vi "MB_TCP_7051.vi"(5 "Status Reference":T1, 6 "N":i32, 7 "Data Reference":T2, 9 "timeouts":T3={"conn_timeout"=1000, "reconn_timeout"=3000, "N attempt max"=3, "t_reset_TTL"=120000, "write_timeout"=10, "read_timeout"=500, "period"=100} {"t_reset_TTL" min=10 max=240000 step=1; "period" min=10 max=100000 step=1; "read_timeout" min=10 max=60000 step=1; "write_timeout" min=1 max=60000 step=1; "N attempt max" min=1 max=5 step=1; "reconn_timeout" min=10 max=240000 step=1; "conn_timeout" min=10 max=240000}, 10 "write enable":bool=TRUE, 11 "stop":bool) -> (0 "error out":errorcluster, 2 "errors":i32, 3 "Z3":u32)   [LabVIEW 2019, in "MB_TCP1.lvlib"]
uses:
  MB_TCP1.lvlib
  Timer Delay/Timers.lvlib
  NI_modbus_upd/NI_modbus_upd.lvlib
  NI_modbus_upd/MB Modbus Command.ctl
  ICPCON Registers/ICPCON Registers.lvlib
  ICPCON Status/ICPCON Status.lvlib
  Timer Delay/unix time 1ms.vi
  NI_modbus_upd/TCP/TCP.lvclass
  ICPCON Registers/Ctl/ICPCON Data.ctl
  ICPCON Status/Ctl/ICPCON Status.ctl
panel:
  out "stopped":bool
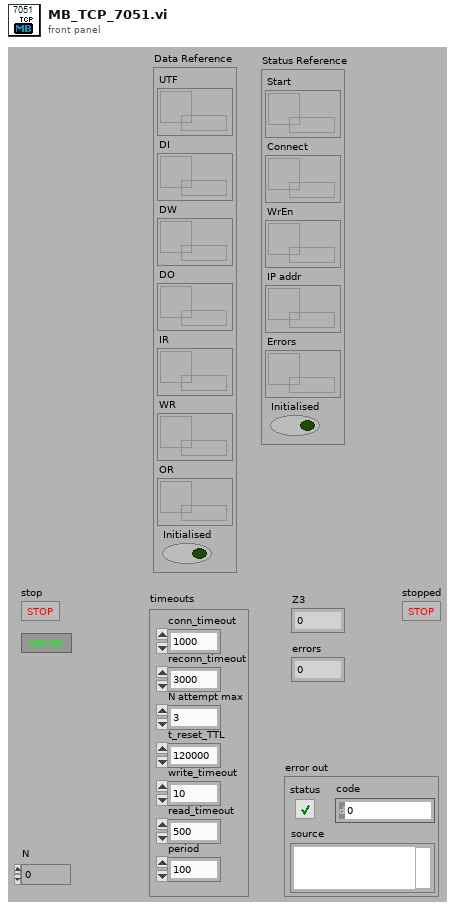
[diagram p1: front panel]
types:
  T1 = typedef "ICPCON Status.lvlib/ICPCON Status.ctl" = cluster{"Start":refnum<data-value>, "Connect":refnum<data-value>, "WrEn":refnum<data-value>, "IP addr":refnum<data-value>, "Errors":refnum<data-value>, "Initialised":bool}
  T2 = typedef "ICPCON Registers.lvlib/ICPCON Data.ctl" = cluster{"UTF":refnum<data-value>, "DI":refnum<data-value>, "DW":refnum<data-value>, "DO":refnum<data-value>, "IR":refnum<data-value>, "WR":refnum<data-value>, "OR":refnum<data-value>, "Initialised":bool}
  T3 = cluster{"conn_timeout":i32, "reconn_timeout":i32, "N attempt max":i32, "t_reset_TTL":i32, "write_timeout":i32, "read_timeout":i32, "period":i32}
  T4 = typedef "NI_modbus_upd.lvlib/MB Modbus Command.ctl" = cluster{"Function Code":u8, "Starting Address":u16, "Quantity":u16, "Data":u16[], "Discrete":bool[]}
  T5 = cluster{"Transaction ID":u16, "Protocol ID":u16, "Length":u16, "Unit ID":u8}
  T6 = cluster{"Remote IP Address":string, "Remote Port":u16}
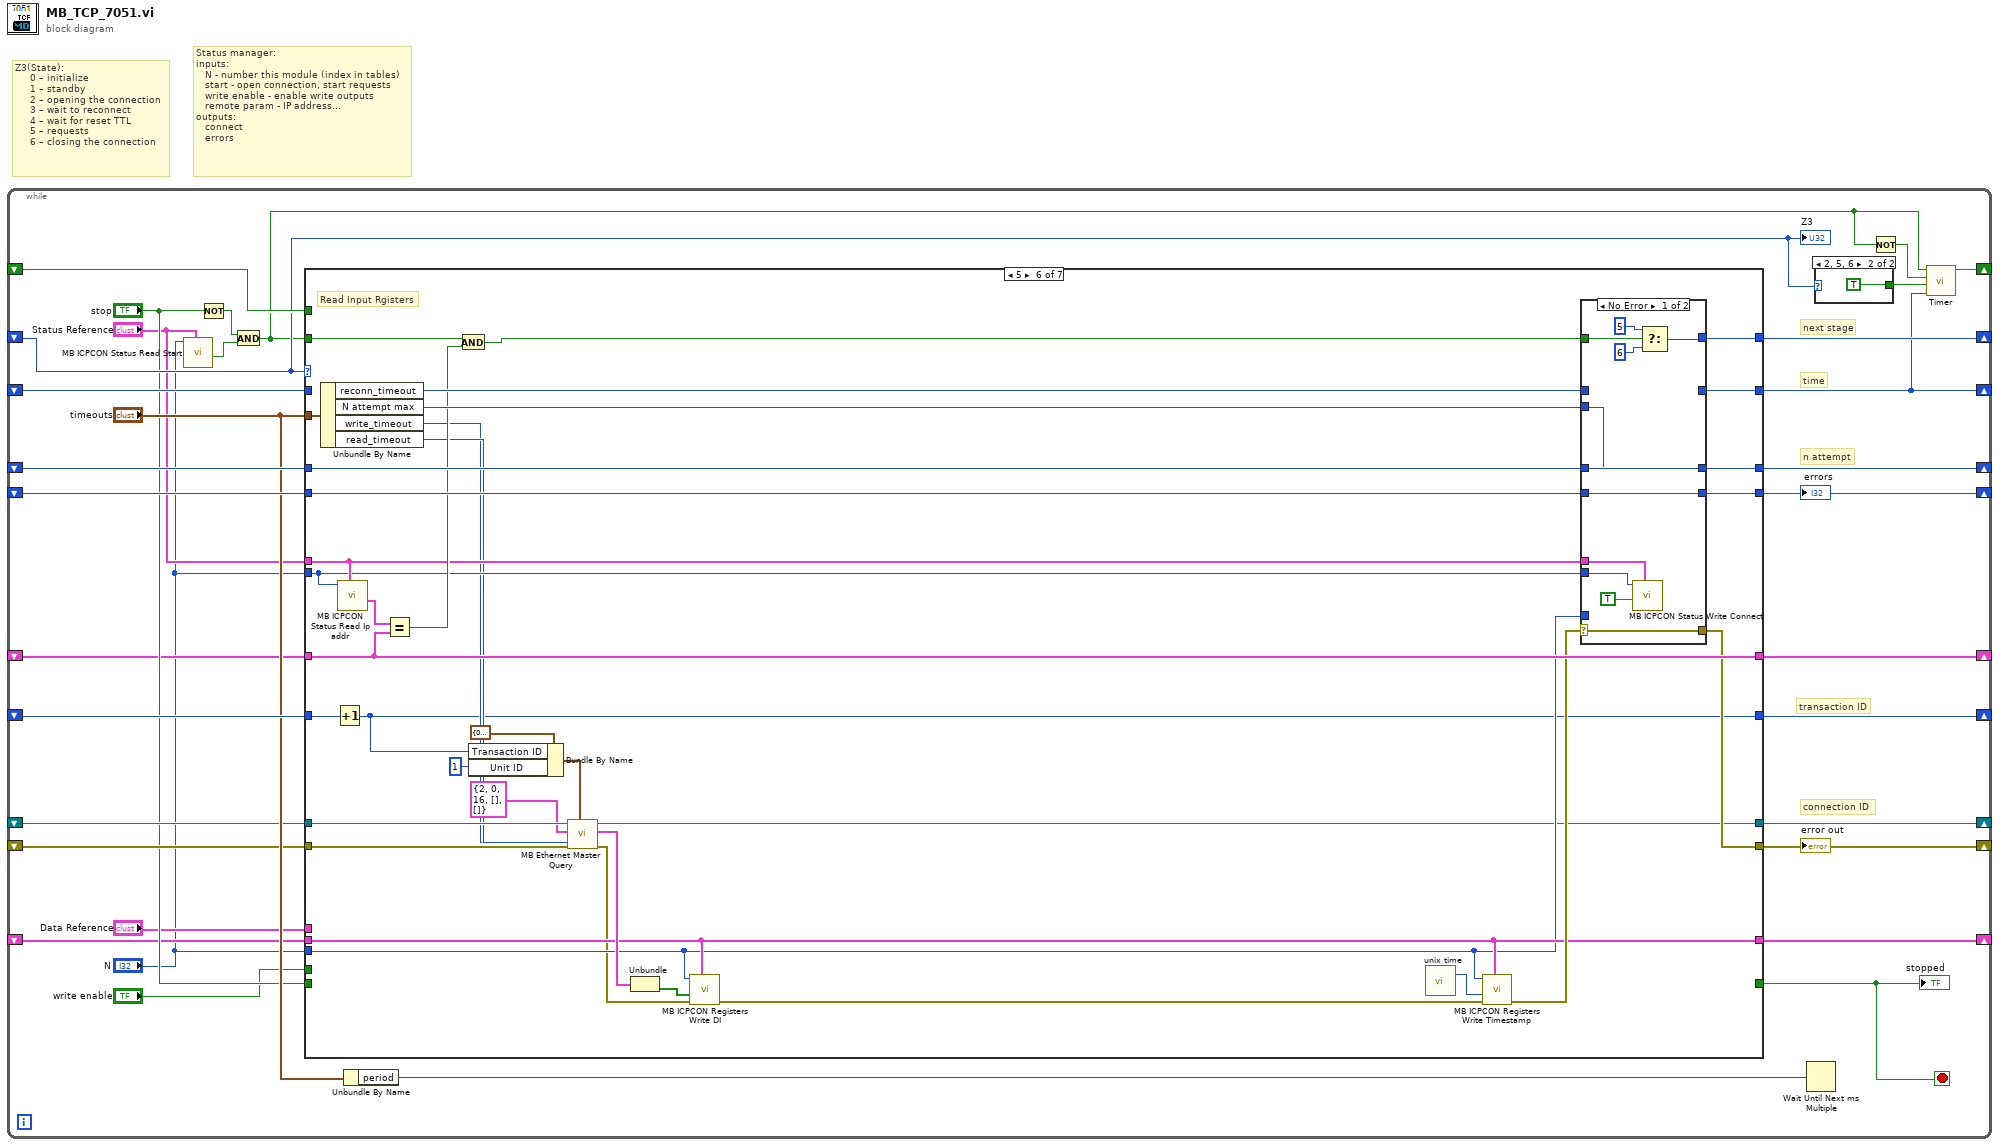
[diagram p0: block diagram]
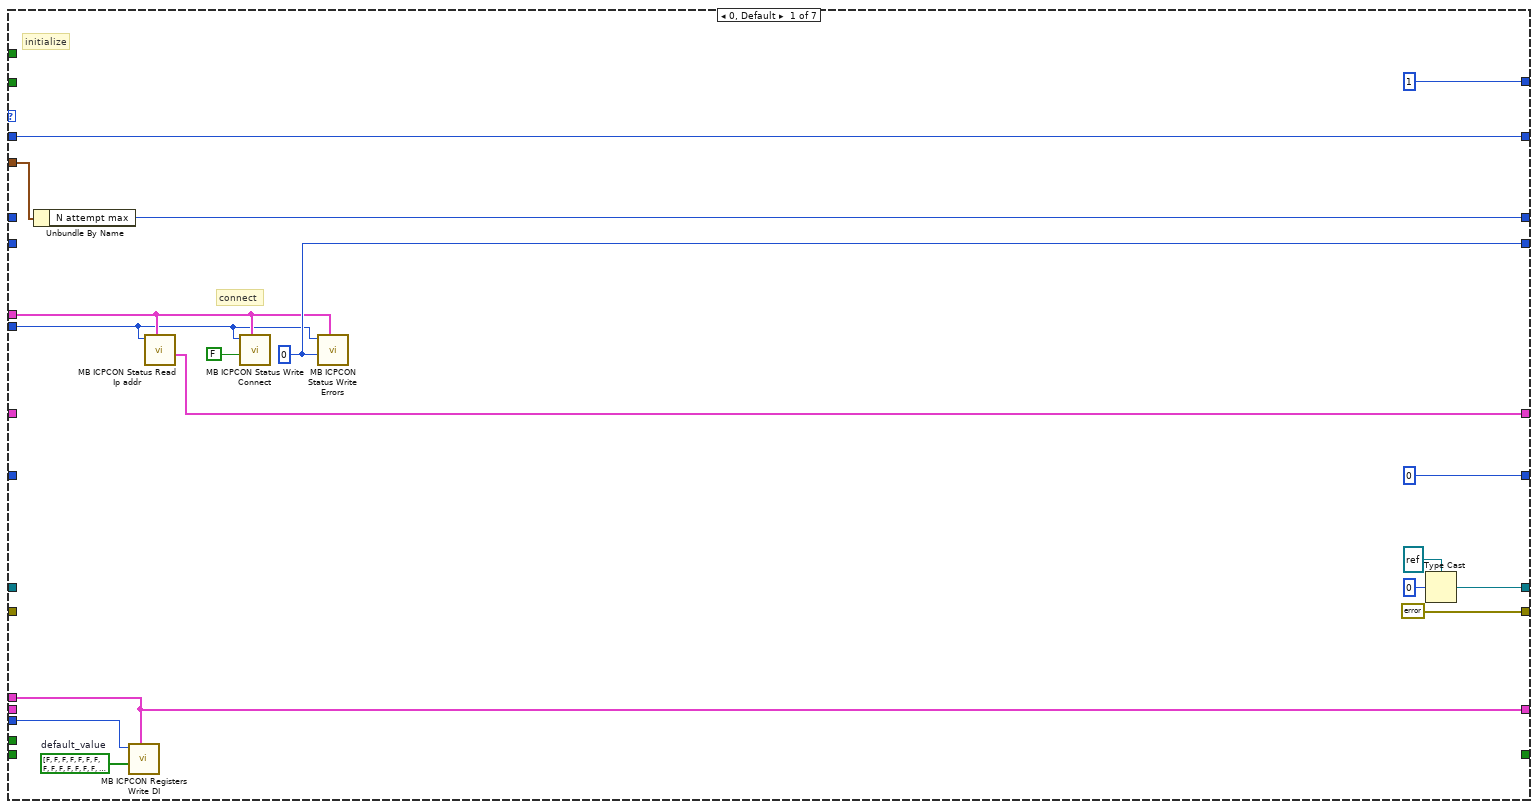
[diagram p2: hidden frame]
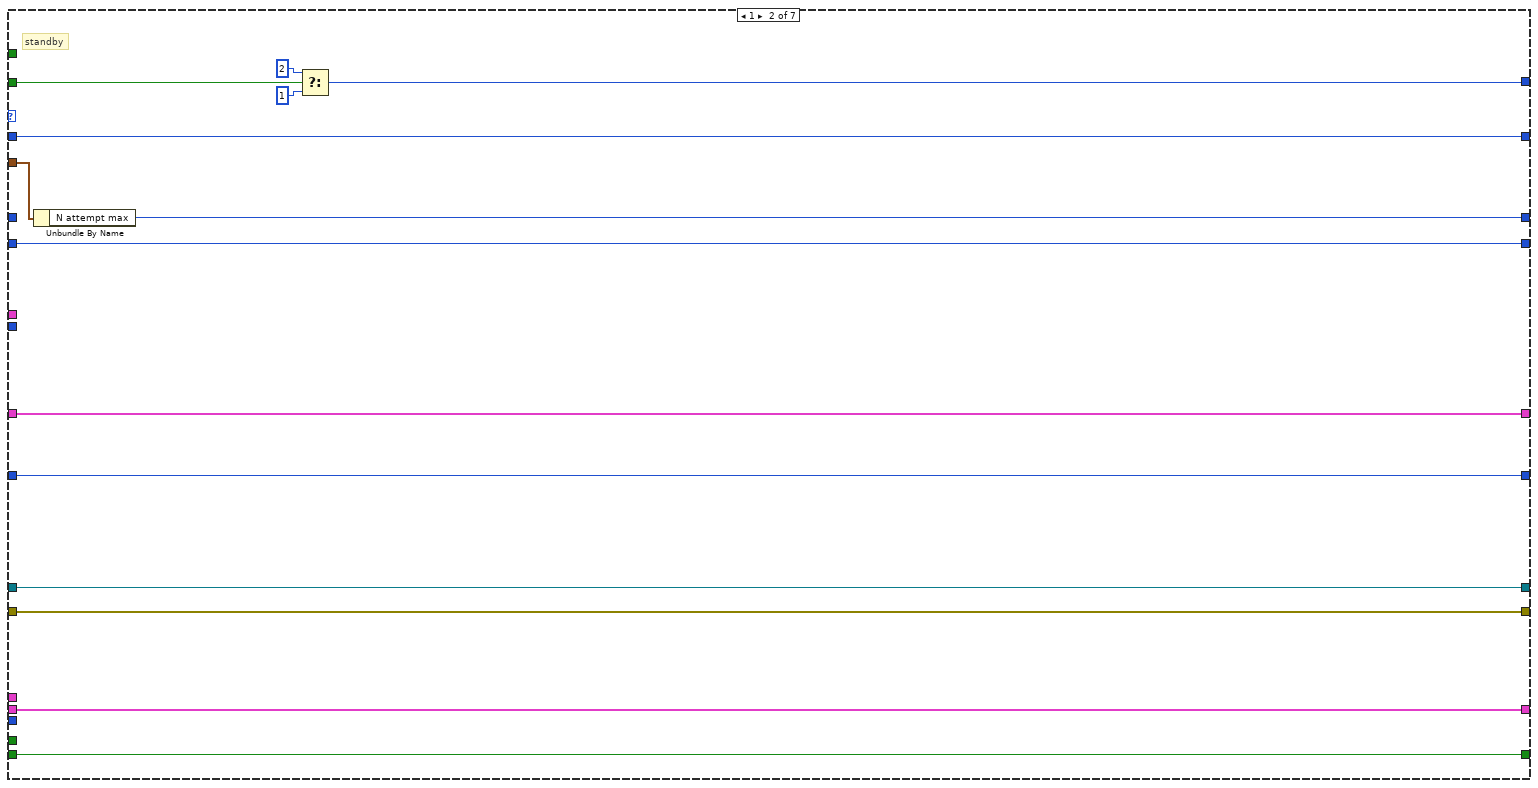
[diagram p3: hidden frame]
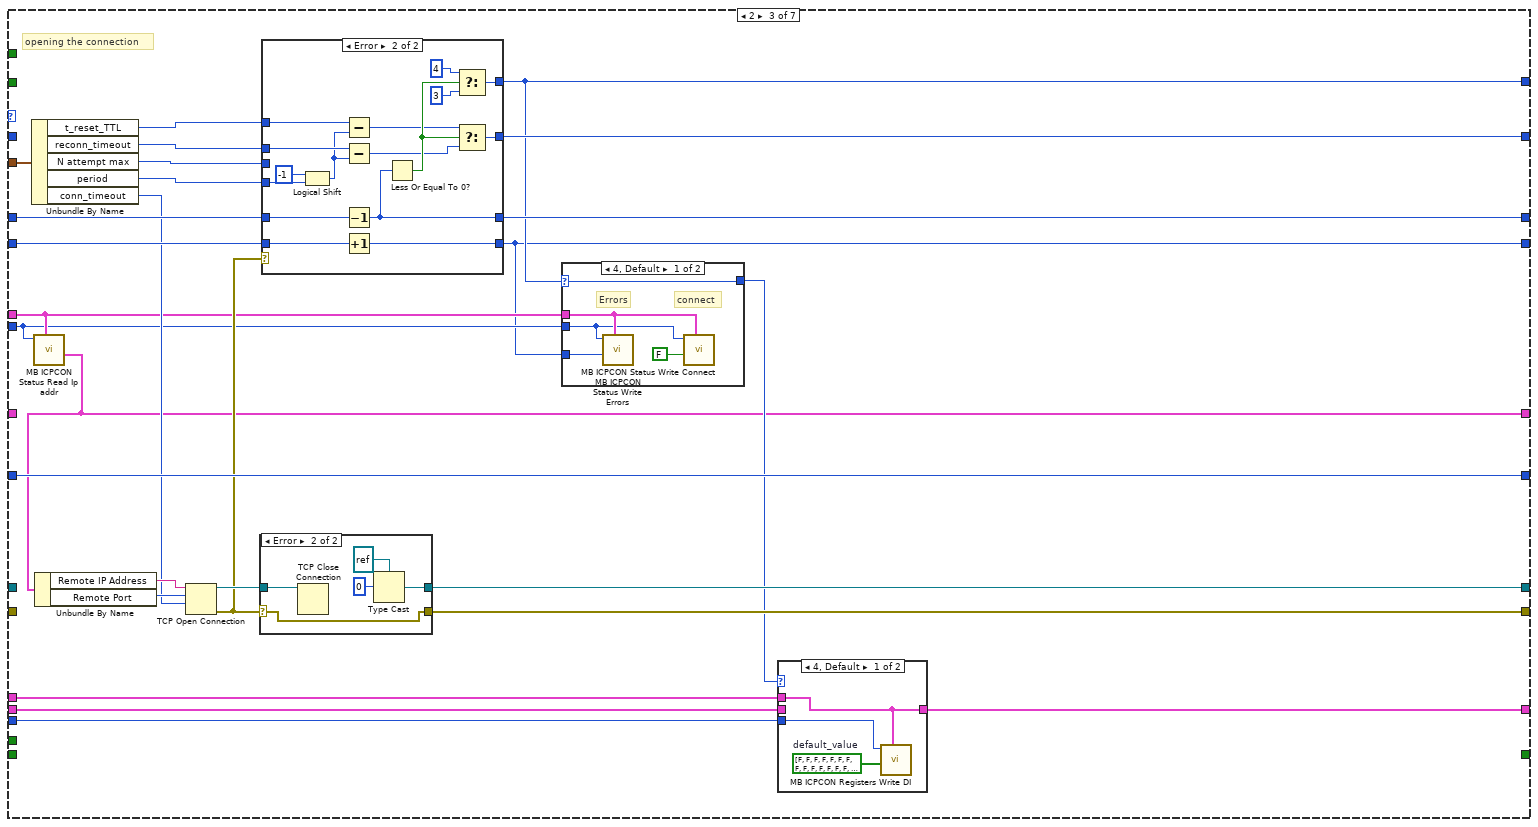
[diagram p4: hidden frame]
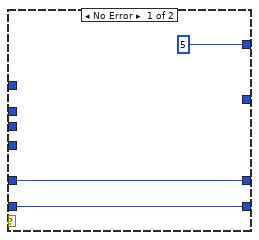
[diagram p8: hidden frame]
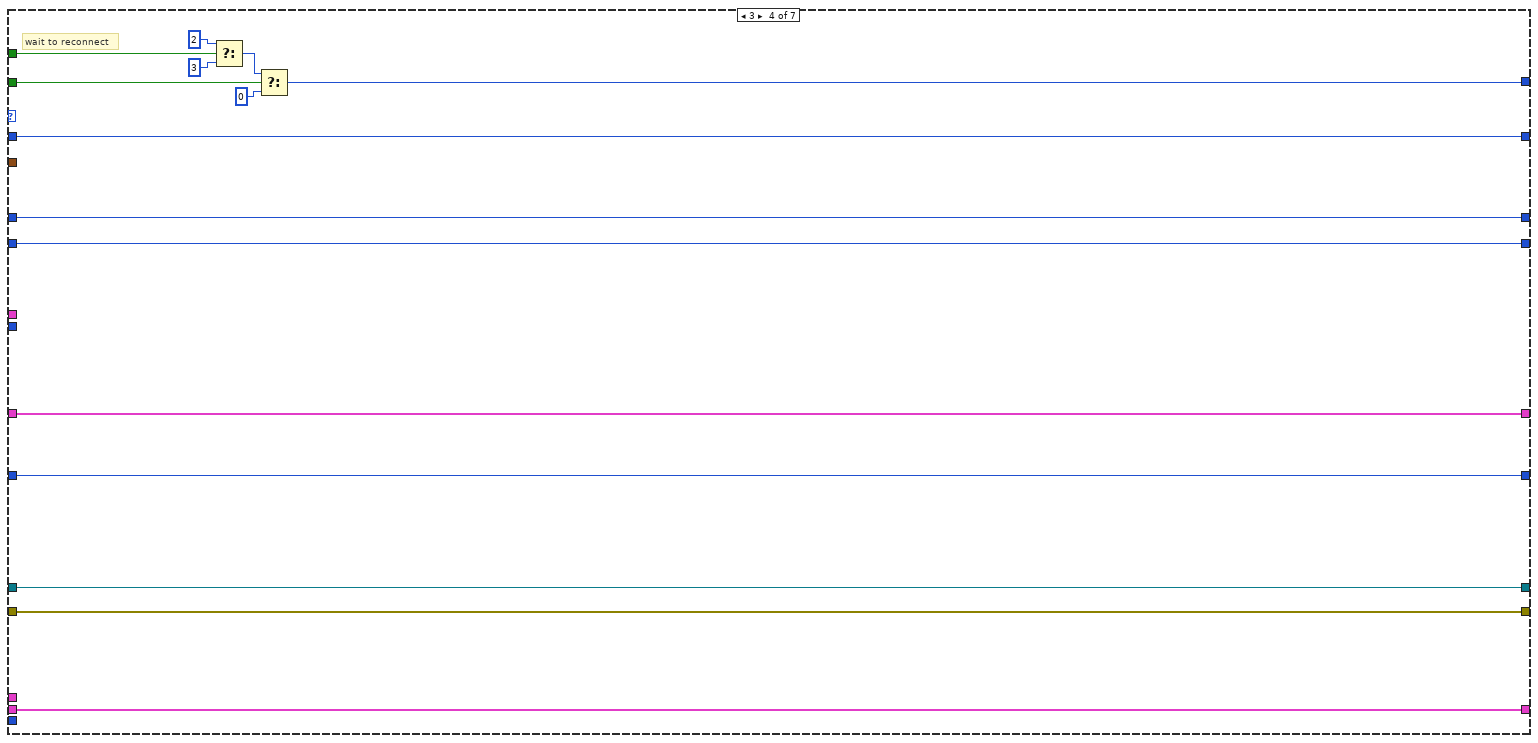
[diagram p9: hidden frame]
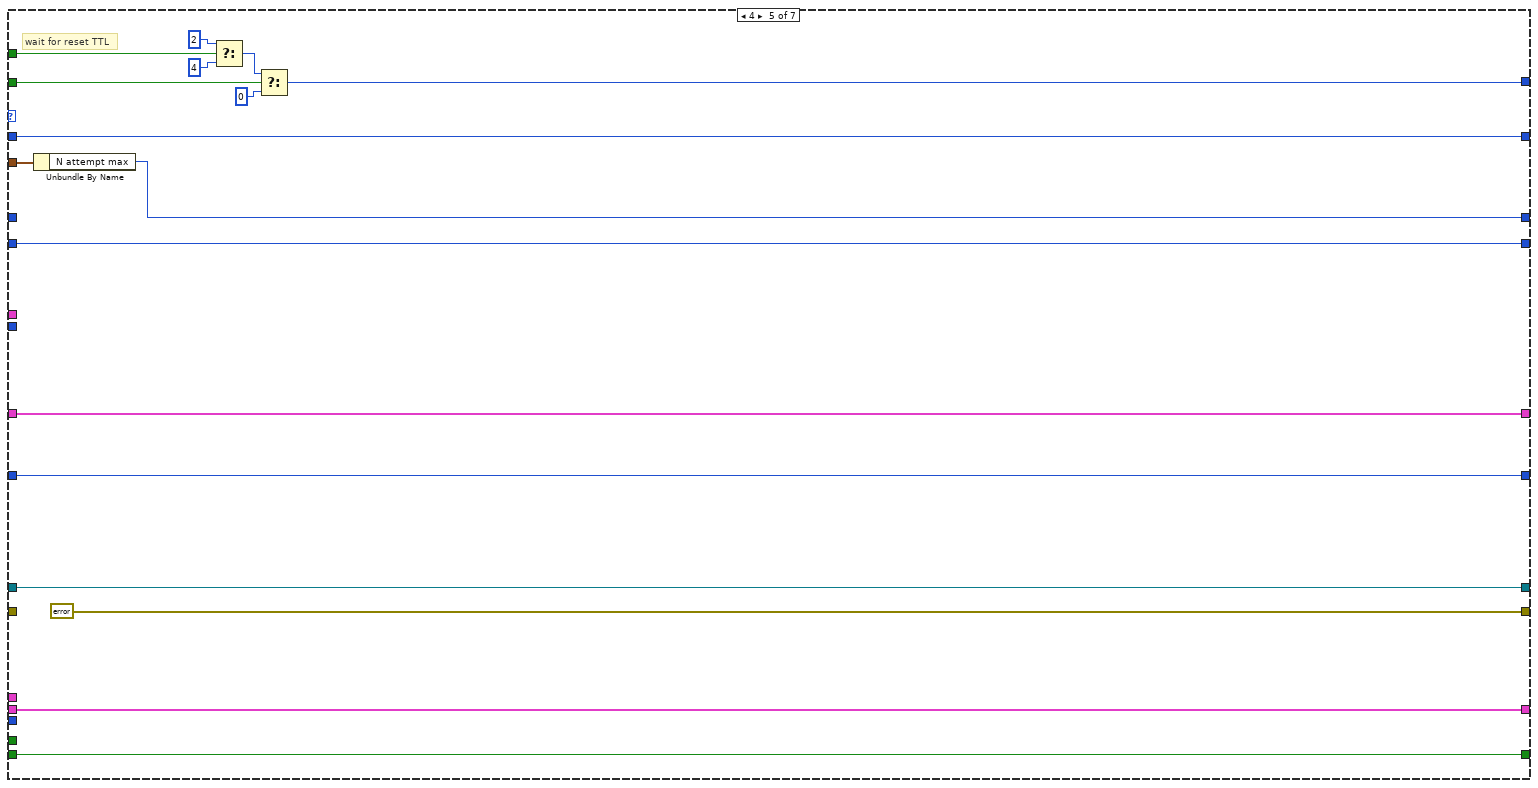
[diagram p10: hidden frame]
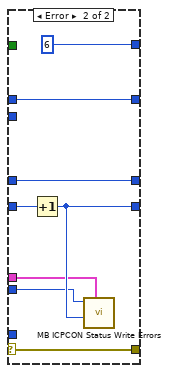
[diagram p11: hidden frame]
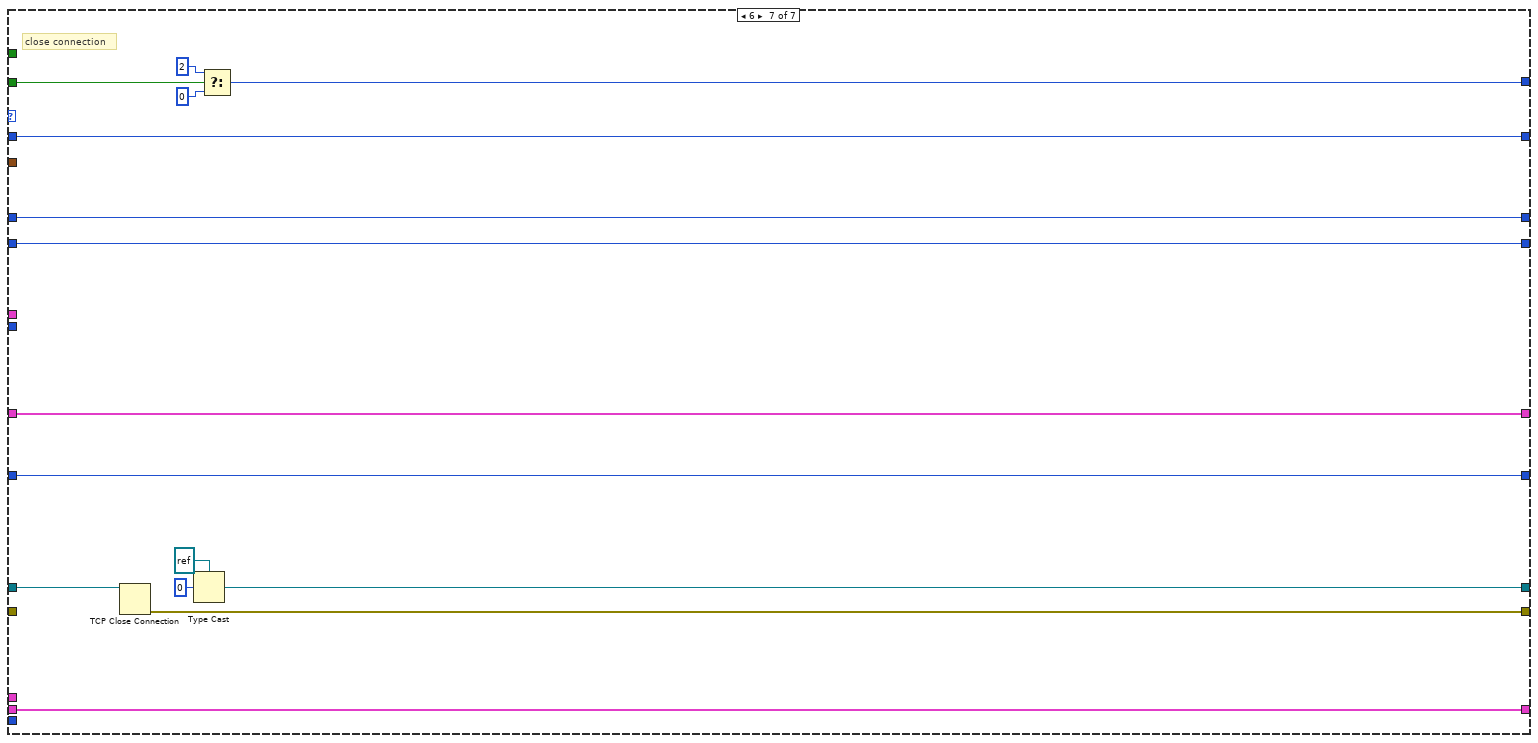
[diagram p12: hidden frame]
diagram:
  # "Status manager:\ninputs:\n   N - number this module (index in tables)\n   start - open connection, start requests\n   write enable - enable write outputs\n   remote param - IP address...\noutputs:\n   connect\n   errors"
  # "Z3(State):\n     0 – initialize \n     1 – standby\n     2 – opening the connection\n     3 – wait to reconnect\n     4 – wait for reset TTL\n     5 – requests\n     6 – closing the connection"
  n1 = while {
    shift-right: [w18] -> _
    shift-left: _ -> [w14]
    shift-right: [w17] -> _
    shift-left: _ -> [w32]
    shift-right: [w31] -> _
    shift-left: _ -> [w29]
    shift-right: [w30] -> _
    shift-left: _ -> [w28]
    shift-right: [w27] -> _
    shift-left: _ -> [w19]
    shift-right: [w26] -> _
    shift-left: _ -> [w20]
    shift-right: [w25] -> _
    shift-left: _ -> [w24]
    shift-right: [w16] -> _
    shift-left: _ -> [w15]
    shift-right: [w10] -> _
    shift-left: _ -> [w9]
    shift-right: [w7] -> _
    shift-left: _ -> [w6]
    stop <- w1 stop-if-true
    # "connection ID"
    # "transaction ID"
    # "n attempt"
    # "time"
    # "next stage"
    n2 = call "MB ICPCON Status Read Start.vi"("Status Reference"="Status Reference", "N"="N") -> ("Start"=w4:bool)  [unwired: 8 in, 1 out]
    n3 = Not(x="stop") -> (.not. x?=w12:bool)
    n4 = And(x=w12, y=w4) -> (x .and. y?=w13:bool)
    n5 = case shown="5" w14 {
      tunnel: [w48 w56 w77 w140 w145 w163 w225] -> w27
      tunnel: [errorcluster {"status"=FALSE, "code"=0, "source"=""} ("error out") w55 w75 w139 errorcluster {"status"=FALSE, "code"=0, "source"=""} ("error out") w175 w226] -> w26
      tunnel: w19 -> [_ w56 _ w140 w145 w185 w222]
      tunnel: w20 -> [_ w55 _ w139 _ w184 _]
      tunnel: w24 -> [_ w64 w91 w142 w159 w194 w227]
      tunnel: [u16 0 ("x") w64 w91 w142 w159 w161 w227] -> w25
      tunnel: [w43 w60 w87 w141 w155 w192 w219] -> w31
      tunnel: w29 -> [_ _ w88 w141 _ w192 w219]
      tunnel: [w40 w63 w65 w138 w158 w191 w224] -> w30
      tunnel: w28 -> [_ w63 w90 w138 w158 w190 w224]
      tunnel: [w45 w62 w84 w137 w157 w187 w223] -> w17
      tunnel: w32 -> [w45 w62 _ w137 w157 _ w223]
      tunnel: "timeouts" -> [w44 w61 w89 _ w156 w193 _]
      tunnel: w13 -> [_ w54 _ w133 w147 w179 w220]
      tunnel: [u32 1 w57 w74 w130 w150 w186 w215] -> w18
      tunnel: w15 -> [_ _ _ w131 w149 _ _]
      tunnel: "N" -> [w36 _ w71 _ _ w166 _]
      tunnel: "stop" -> [_ w53 _ _ w146 _ _]
      tunnel: [_ w53 _ _ w146 _ _] -> w1
      tunnel: [w41 w52 w68 w129 w144 w177 w214] -> w10
      tunnel: w9 -> [_ w52 _ w129 w144 w177 w214]
      tunnel: "Data Reference" -> [w37 _ w70 _ _ _ _]
      tunnel: [w37 w51 w73 w128 w143 w167 w213] -> w7
      tunnel: w6 -> [_ w51 w69 w128 w143 w167 w213]
      tunnel: "write enable" -> [_ _ _ _ _ _ _]
      tunnel: "Status Reference" -> [w39 _ w67 _ _ w171 _]
      tunnel: "N" -> [w38 _ w66 _ _ w170 _]
      frame 0, Default {
        w40 = 0 ("N attempt max")
        w35 = bool[] [FALSE, FALSE, FALSE, FALSE, FALSE, FALSE, FALSE, FALSE, FALSE, FALSE, FALSE, FALSE, FALSE, FALSE, FALSE, FALSE, FALSE, FALSE, FALSE, FALSE, FALSE, FALSE, FALSE, FALSE, FALSE, FALSE, FALSE, FALSE, FALSE, FALSE, FALSE, FALSE]  # default_value
        # "connect"
        # "initialize"
        n6 = Unbundle By Name(w44) -> ("N attempt max"=w43:i32)
        n7 = call "MB ICPCON Registers Write DI.vi"("Data Reference"=w37, "Bits In"=w35, "N"=w36) -> ()  [unwired: 8 in, 1 out]
        n8 = call "MB ICPCON Status Read Ip addr.vi"("Status Reference"=w39, "N"=w38) -> ("IP address"=w41:T6)  [unwired: 8 in, 1 out]
        n9 = call "MB ICPCON Status Write Connect.vi"("Status Reference"=w39, "Connect"=FALSE ("connect"), "N"=w38) -> ()  [unwired: 8 in, 1 out]
        n10 = call "MB ICPCON Status Write Errors.vi"("Status Reference"=w39, "Errors"=w40, "N"=w38) -> ()  [unwired: 8 in, 1 out]
        n11 = Type Cast(type=refnum<k5> refnum ("connection ID"), x=u32 0) -> (*(type *) &x=w48:refnum<k5>)
      }
      frame 1 {
        # "standby"
        n12 = Unbundle By Name(w61) -> ("N attempt max"=w60:i32)
        n13 = Select(t=u32 2, s=w54, f=u32 1) -> (s? t:f=w57:u32)
      }
      frame 2 {
        # "opening the connection"
        n14 = Unbundle By Name(w89) -> ("t_reset_TTL"=w83:i32, "reconn_timeout"=w85:i32, "N attempt max"=w86:i32, "period"=w80:i32, "conn_timeout"=w79:i32)
        n15 = call "MB ICPCON Status Read Ip addr.vi"("Status Reference"=w67, "N"=w66) -> ("IP address"=w68:T6)  [unwired: 8 in, 1 out]
        n16 = Unbundle By Name(w68) -> ("Remote IP Address"=w82:string, "Remote Port"=w81:u16)
        n17 = TCP Open Connection(address=w82, remote port or service name=w81, timeout ms (60000)=w79) -> (connection ID=w78:refnum<k5>, error out=w76:errorcluster)  [unwired: 2 in]
        n18 = case shown="Error" w76 {
          selector: w76 -> [w102 w104]
          tunnel: w78 -> [w103 w107]
          tunnel: [w103 w106] -> w77
          tunnel: [w102 w104] -> w75
          frame No Error {
          }
          frame Error {
            n19 = TCP Close Connection(connection ID=w107) -> ()  [unwired: 2 in, 2 out]
            n20 = Type Cast(type=refnum<k5> refnum ("connection ID"), x=u32 0) -> (*(type *) &x=w106:refnum<k5>)
          }
        }
        n21 = case shown="Error" w76 {
          tunnel: w90 -> [w111 w127]
          tunnel: [w111 w126] -> w65
          tunnel: w88 -> [w110 w125]
          tunnel: [w110 w124] -> w87
          tunnel: w86 -> [_ _]
          tunnel: [u32 5 w121] -> w74
          tunnel: w85 -> [_ w120]
          tunnel: [_ w119] -> w84
          tunnel: w83 -> [_ w116]
          tunnel: w80 -> [_ w114]
          frame No Error {
          }
          frame Error {
            n22 = Logical Shift(y=i16 -1, x=w114) -> (x << y=w112:i32)
            n23 = Subtract(x=w116, y=w112) -> (x-y=w115:i32)
            n24 = Subtract(x=w120, y=w112) -> (x-y=w117:i32)
            n25 = Decrement(x=w125) -> (x-1=w124:i32)
            n26 = Increment(x=w127) -> (x+1=w126:i32)
            n27 = Less Or Equal To 0?(x=w124) -> (x <= 0?=w118:bool)
            n28 = Select(t=u32 4, s=w118, f=u32 3) -> (s? t:f=w121:u32)
            n29 = Select(t=w115, s=w118, f=w117) -> (s? t:f=w119:i32)
          }
        }
        n30 = case shown="4, Default" w74 {
          selector: w74 -> [w100 w101]
          tunnel: [w100 w101] -> w72
          tunnel: w67 -> [w99 _]
          tunnel: w66 -> [w98 _]
          tunnel: w65 -> [w97 _]
          frame 4, Default {
            # "Errors"
            # "connect"
            n31 = call "MB ICPCON Status Write Errors.vi"("Status Reference"=w99, "Errors"=w97, "N"=w98) -> ()  [unwired: 8 in, 1 out]
            n32 = call "MB ICPCON Status Write Connect.vi"("Status Reference"=w99, "Connect"=FALSE ("f"), "N"=w98) -> ()  [unwired: 8 in, 1 out]
          }
          frame 3, 5 {
          }
        }
        n33 = case shown="4, Default" w72 {
          tunnel: w71 -> [w94 _]
          tunnel: w69 -> [_ w95]
          tunnel: [w93 w95] -> w73
          tunnel: w70 -> [w93 _]
          frame 4, Default {
            w92 = bool[] [FALSE, FALSE, FALSE, FALSE, FALSE, FALSE, FALSE, FALSE, FALSE, FALSE, FALSE, FALSE, FALSE, FALSE, FALSE, FALSE, FALSE, FALSE, FALSE, FALSE, FALSE, FALSE, FALSE, FALSE, FALSE, FALSE, FALSE, FALSE, FALSE, FALSE, FALSE, FALSE]  # default_value
            n34 = call "MB ICPCON Registers Write DI.vi"("Data Reference"=w93, "Bits In"=w92, "N"=w94) -> ()  [unwired: 8 in, 1 out]
          }
          frame 3, 5 {
          }
        }
      }
      frame 3 {
        # "wait to reconnect"
        n35 = Select(t=u32 2, s=w131, f=u32 3) -> (s? t:f=w132:u32)
        n36 = Select(t=w132, s=w133, f=u32 0) -> (s? t:f=w130:u32)
      }
      frame 4 {
        # "wait for reset TTL"
        n37 = Unbundle By Name(w156) -> ("N attempt max"=w155:i32)
        n38 = Select(t=u32 2, s=w149, f=u32 4) -> (s? t:f=w151:u32)
        n39 = Select(t=w151, s=w147, f=u32 0) -> (s? t:f=w150:u32)
      }
      frame 5 {
        # "Read Input Rgisters"
        n40 = Unbundle By Name(w193) -> ("reconn_timeout"=w188:i32, "N attempt max"=w189:i32, "write_timeout"=w164:i32, "read_timeout"=w168:i32)
        n41 = Increment(x=w194) -> (x+1=w161:u16)
        n42 = call "MB ICPCON Status Read Ip addr.vi"("Status Reference"=w171, "N"=w170) -> ("IP address"=w172:T6)  [unwired: 8 in, 1 out]
        n43 = Equal?(x=w172, y=w177) -> (x = y?=w176:bool)
        n44 = And(x=w179, y=w176) -> (x .and. y?=w178:bool)
        n45 = Bundle By Name(cluster=T5 {"Transaction ID"=0, "Protocol ID"=0, "Length"=0, "Unit ID"=0} ("MBAP Header"), "Transaction ID"=w161, "Unit ID"=u8 1) -> (w180:T5)
        n46 = call "MB Ethernet Master Query.vi"(4:w168, 6:w164, "MBAP Header"=w180, "error in (no error)"=w184, "Modbus Command"=T4 {"Function Code"=2, "Starting Address"=0, "Quantity"=16, "Data"=[], "Discrete"=[]}, "TCP in"=w185) -> ("error out"=w162:errorcluster, "Registers"=w183:cluster{"Registers":u16[], "Discrete":bool[]}, "TCP out"=w163:refnum<class "TCP.lvclass">)  [unwired: 2 in, 1 out]
        n47 = Unbundle(w183) -> ("Discrete"=w160:bool[])  [unwired: 1 out]
        n48 = call "MB ICPCON Registers Write DI.vi"("Data Reference"=w167, "error in (no error)"=w162, "Bits In"=w160, "N"=w166) -> ("error out"=w165:errorcluster)  [unwired: 7 in]
        n49 = call-poly "unix time.vi"() -> ("unix time (ms)"=w173:u64)  [unwired: 2 in, 1 out]
        n50 = call "MB ICPCON Registers Write Timestamp.vi"("Data Reference"=w167, "error in (no error)"=w165, "UTF"=w173, "N"=w166) -> ("error out"=w174:errorcluster)  [unwired: 7 in]
        n51 = case shown="No Error" w174 {
          selector: w174 -> [w198 w208]
          tunnel: w190 -> [w199 w212]
          tunnel: [w199 w207] -> w191
          tunnel: [w201 u32 6] -> w186
          tunnel: w192 -> [_ w210]
          tunnel: w189 -> [w204 _]
          tunnel: [w204 w210] -> _
          tunnel: w188 -> [_ w209]
          tunnel: [_ w209] -> w187
          tunnel: w178 -> [w200 _]
          tunnel: w166 -> [_ _]
          tunnel: [w198 w208] -> w175
          tunnel: w171 -> [w197 w206]
          tunnel: w170 -> [w196 w205]
          frame No Error {
            n52 = call "MB ICPCON Status Write Connect.vi"("Status Reference"=w197, "Connect"=TRUE ("f"), "N"=w196) -> ()  [unwired: 8 in, 1 out]
            n53 = Select(t=u32 5, s=w200, f=u32 6) -> (s? t:f=w201:u32)
          }
          frame Error {
            n54 = Increment(x=w212) -> (x+1=w207:i32)
            n55 = call "MB ICPCON Status Write Errors.vi"("Status Reference"=w206, "Errors"=w207, "N"=w205) -> ()  [unwired: 8 in, 1 out]
          }
        }
      }
      frame 6 {
        # "close connection"
        n56 = TCP Close Connection(connection ID=w222) -> (error out=w226:errorcluster)  [unwired: 2 in, 1 out]
        n57 = Type Cast(type=refnum<k5> refnum ("connection ID"), x=u32 0) -> (*(type *) &x=w225:refnum<k5>)
        n58 = Select(t=u32 2, s=w220, f=u32 0) -> (s? t:f=w215:u32)
      }
    }
    "error out" <- w26
    "errors" <- w30
    "stopped" <- w1
    n59 = Unbundle By Name("timeouts") -> ("period"=w22:i32)
    n60 = Wait Until Next ms Multiple(millisecond multiple=w22) -> ()  [unwired: 1 out]
    n61 = case shown="2, 5, 6" w14 {
      tunnel: [_ TRUE] -> w21
      frame 0, Default {
      }
      frame 2, 5, 6 {
      }
    }
    n62 = Not(x=w13) -> (.not. x?=w33:bool)
    n63 = call "Timer.vi"("ms"=w17, "Load (F)"=w21, "Reset (F)"=w33, "Start (T)"=w13) -> ("End"=w16:bool)  [unwired: 5 in, 1 out]
    "Z3" <- w14
  }
